vi "Create Industrial Controller.vi"(8 "error in (no error)":errorcluster, 10 "Settings":T3, 11 "Custom Device Ref":refnum<k24>) -> (0 "error out":errorcluster, 3 "Custom Device Ref":refnum<k24>)   [LabVIEW 2013, in "Control SysDef API.lvlib"]
uses:
  Control SysDef API.lvlib
  NationalInstruments.VeriStand.SystemDefinitionAPI
  Shared/Types/Controller Settings.ctl
  Shared/Types/Industrial Parameters.ctl
  Shared/Types/Action.ctl
  Shared/Constants.vi
  <vilib>/NI Veristand/Custom Device API/NI VeriStand - Set Item Property.vi
  <vilib>/NI Veristand/Custom Device API/Set Item Property (Double).vi
  <vilib>/NI Veristand/Custom Device API/Set Item Property (Boolean).vi
  <vilib>/NI Veristand/Custom Device Tools/Custom Device Utility Library/NI VeriStand - Search for Item.vi
  <vilib>/NI Veristand/Custom Device Tools/Custom Device Utility Library/NI VeriStand - Search for Item by GUID.vi
  <vilib>/NI Veristand/Custom Device API/NI VeriStand - Add Custom Device Channel.vi
  <vilib>/NI Veristand/Custom Device API/NI VeriStand - Remove Custom Device Item.vi
  Shared/Control Addon Shared.lvlib
  <vilib>/NI Veristand/Custom Device API/Custom Device API.lvlib
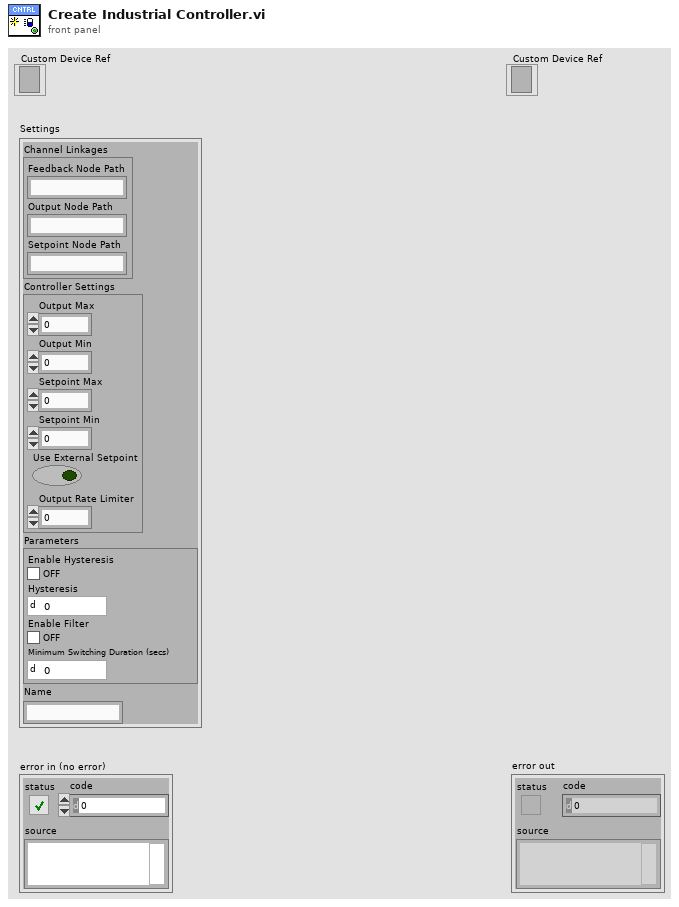
[diagram p1: front panel]
types:
  T1 = typedef "Control Addon Shared.lvlib/Controller Settings.ctl" = cluster{"Output Max":dbl, "Output Min":dbl, "Setpoint Max":dbl, "Setpoint Min":dbl, "Use External Setpoint":bool, "Output Rate Limiter":dbl}
  T2 = typedef "Control Addon Shared.lvlib/Industrial Parameters.ctl" = cluster{"Enable Hysteresis":bool, "Hysteresis":dbl, "Enable Filter":bool, "Minimum Switching":dbl}
  T3 = cluster{"Channel Linkages":cluster{"Feedback Node Path":string, "Output Node Path":string, "Setpoint Node Path":string}, "Controller Settings":T1, "Parameters":T2, "Name":string}
  T4 = typedef "Control Addon Shared.lvlib/Action.ctl" = enum16{"Get", "Set"}
  T5 = typedef "Custom Device API.lvlib/Custom Device Item Ref.ctl" = u64
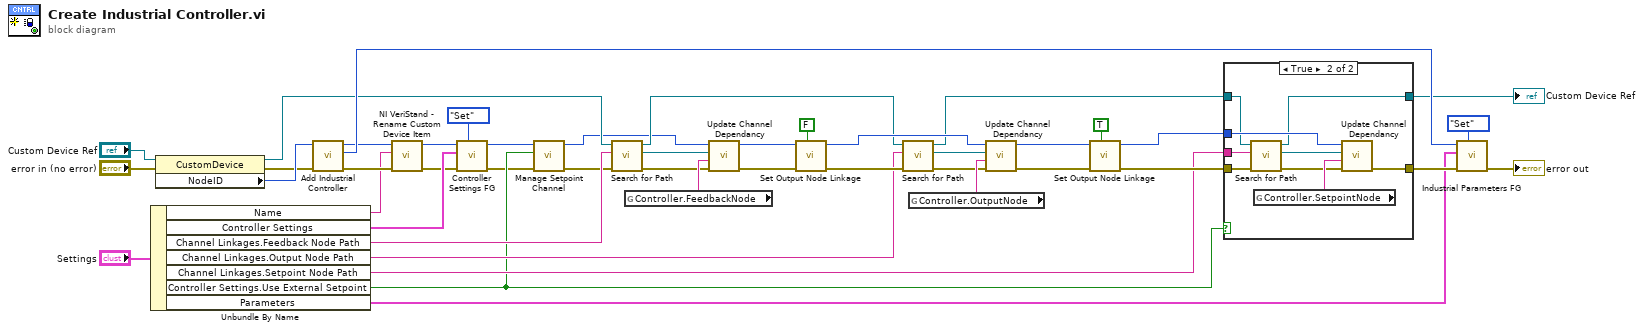
[diagram p0: block diagram]
diagram:
  n1 = Unbundle By Name("Settings") -> ("Name"=w6:string, "Controller Settings"=w12:T1, "Channel Linkages.Feedback Node Path"=w24:string, "Channel Linkages.Output Node Path"=w19:string, "Channel Linkages.Setpoint Node Path"=w16:string, "Controller Settings.Use External Setpoint"=w5:bool, "Parameters"=w11:T2)
  n2 = property class="CustomDevice"(reference="Custom Device Ref", error in="error in (no error)") -> (reference out=w25:refnum<k24>, error out=w27:errorcluster, "NodeID"=w43:u64)
  n3 = call "Add Industrial Controller.vi"("error in (no error)"=w27, "Node Ptr"=w43) -> ("error out"=w9:errorcluster, "Parameters Ref out"=w30:T5, "Controller Ref out"=w8:T5)  [unwired: 7 in]
  n4 = call <vilib>:"NI VeriStand - Rename Custom Device Item.vi"("error in (no error)"=w9, "New Name"=w6, "Item Ref in"=w8) -> ("error out"=w10:errorcluster, "Item Ref out"=w7:T5)  [unwired: 6 in, 1 out]
  n5 = call "Controller Settings FG.vi"("Action"=Action."Set", "error in (no error)"=w10, "Controller Settings"=w12, "Node Ptr"=w7) -> ("error out"=w3:errorcluster, "Item Ref out"=w4:T5)  [unwired: 5 in, 1 out]
  n6 = call "Manage Setpoint Channel.vi"("error in (no error)"=w3, "Use External Setpoint"=w5, "Node Ptr"=w4) -> ("error out"=w2:errorcluster, "Node Ptr out"=w1:T5)  [unwired: 7 in]
  n7 = call "Search for Path.vi"("error in (no error)"=w2, "nodepath"=w24, "Custom Device Ref"=w25) -> ("error out"=w26:errorcluster, "BaseNodeType"=w23:refnum<k24>, "Custom Device Ref"=w20:refnum<k24>)  [unwired: 6 in]
  n8 = global read "Constants.vi" "Controller.FeedbackNode"() -> (w40:string)
  n9 = call "Update Channel Dependancy.vi"("error in (no error)"=w26, "NodeName"=w40, "Data"=w23, "Item Ref in"=w1) -> ("error out"=w35:errorcluster, "Item Ref out"=w34:T5)  [unwired: 6 in]
  n10 = call "Set Output Node Linkage.vi"("Add?"=FALSE, "error in"=w35, "Section Ref in"=w34) -> ("error out"=w22:errorcluster, "Item Ref out"=w39:T5)  [unwired: 7 in]
  n11 = call "Search for Path.vi"("error in (no error)"=w22, "nodepath"=w19, "Custom Device Ref"=w20) -> ("error out"=w21:errorcluster, "BaseNodeType"=w18:refnum<k24>, "Custom Device Ref"=w15:refnum<k24>)  [unwired: 6 in]
  n12 = global read "Constants.vi" "Controller.OutputNode"() -> (w36:string)
  n13 = call "Update Channel Dependancy.vi"("error in (no error)"=w21, "NodeName"=w36, "Data"=w18, "Item Ref in"=w39) -> ("error out"=w33:errorcluster, "Item Ref out"=w32:T5)  [unwired: 6 in]
  n14 = call "Set Output Node Linkage.vi"("Add?"=TRUE, "error in"=w33, "Section Ref in"=w32) -> ("error out"=w17:errorcluster, "Item Ref out"=w31:T5)  [unwired: 7 in]
  n15 = case shown="True" w5 {
    tunnel: w31 -> [_ w55]
    tunnel: [w46 w54] -> w29
    tunnel: w17 -> [w46 w53]
    tunnel: w16 -> [_ w51]
    tunnel: w15 -> [w47 w50]
    tunnel: [w47 w48] -> w14
    frame False {
    }
    frame True {
      n16 = call "Search for Path.vi"("error in (no error)"=w53, "nodepath"=w51, "Custom Device Ref"=w50) -> ("error out"=w52:errorcluster, "BaseNodeType"=w49:refnum<k24>, "Custom Device Ref"=w48:refnum<k24>)  [unwired: 6 in]
      n17 = global read "Constants.vi" "Controller.SetpointNode"() -> (w56:string)
      n18 = call "Update Channel Dependancy.vi"("error in (no error)"=w52, "NodeName"=w56, "Data"=w49, "Item Ref in"=w55) -> ("error out"=w54:errorcluster)  [unwired: 6 in, 1 out]
    }
  }
  "Custom Device Ref" <- w14
  n19 = call "Industrial Parameters FG.vi"("Action"=Action."Set", "error in (no error)"=w29, "Parameters"=w11, "Node Ptr"=w30) -> ("error out"=→"error out":errorcluster)  [unwired: 5 in, 2 out]
